vi "SUB_ChannelToEnergy.vi"(1 "Intercept":dbl, 2 "Channel":dbl, 3 "Slope":dbl) -> (0 "Energy":dbl)   [LabVIEW 2015]
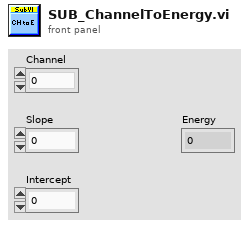
[diagram p1: front panel]
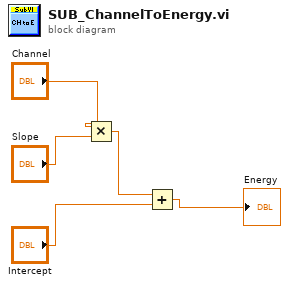
[diagram p0: block diagram]
diagram:
  n1 = Multiply(x="Channel", y="Slope") -> (x*y=w3:dbl)
  n2 = Add(x=w3, y="Intercept") -> (x+y=→"Energy":dbl)
